vi "Get Info.vi"(8 "error in (no error)":errorcluster, 11 "2DPanelBlank in":refnum<class "2DPanelBlank.lvclass">) -> (0 "error out":errorcluster, 2 "Info":T1={"Index"={"Row"=0, "Col"=0}, "State"=enum."Idle"}, 3 "2DPanelBlank out":refnum<class "2DPanelBlank.lvclass">)   [LabVIEW 2020, in "OOPanel.lvlib" / "2DPanelBlank.lvclass"]
uses:
  2DPanelBlank.lvclass
  2DPanelBlank.lvclass/2DPanelBlank.ctl
  2D Index.ctl
  OOPanel.lvlib
  State.ctl
  Info.ctl
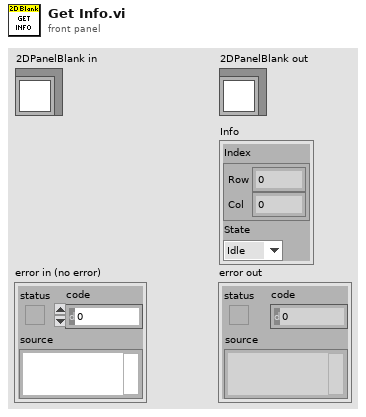
[diagram p1: front panel]
types:
  T1 = typedef "OOPanel.lvlib/2DPanelBlank.lvclass/Info.ctl" = cluster{"Index":T2, "State":T3}
  T2 = typedef "OOPanel.lvlib/2D Index.ctl" = cluster{"Row":i32, "Col":i32}
  T3 = typedef "OOPanel.lvlib/2DPanelBlank.lvclass/State.ctl" = enum16{"New", "Idle", "Pool", "Used"}
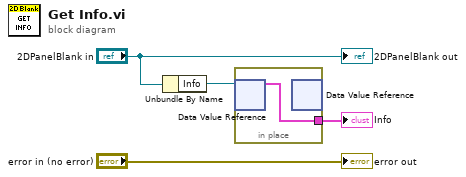
[diagram p0: block diagram]
diagram:
  n1 = Unbundle By Name("2DPanelBlank in") -> ("Info"=w3:refnum<data-value>)
  n2 = in-place {
    in-place-border: [w5] -> w1
    n3 = in-place-dvr #1(w3) -> (w5:T1)  [unwired: 1 out]
    n4 = in-place-dvr #1() -> ()  [unwired: 1 in, 2 out]
  }
  "Info" <- w1
  "error out" <- "error in (no error)"
  "2DPanelBlank out" <- "2DPanelBlank in"
